vi "RegisterPublisher.vi"(6 "Lock Topic":bool, 7 "Topic Name":string, 8 "error in (no error)":errorcluster, 11 "Message Broker Interface Ref in":refnum<class "Message Broker Interface Ref.lvclass">) -> (0 "error out":errorcluster, 2 "Topic Actor Created?":bool, 3 "Message Broker Interface Ref out":refnum<class "Message Broker Interface Ref.lvclass">, 4 "Locked?":bool, 5 "Transport":refnum<class "Message Transport Queue.lvclass">)   [LabVIEW 2016, in "Stream Mediator.lvlib" / "Message Broker Interface Ref.lvclass"]
doc: "--\nCopyright © 2017 Composed SystemsI All rights reserved.\n\nAuthor: Jon McBee <jon.mcbee@composed.io>\n\nThis library is provided \"AS IS\" ,WITHOUT WARRANTIES OR\nCONDITIONS OF ANY KIND, either express or implied.\n\nComposed Systems -- composed.io\n\nStream 0.0.1.1\nJon McBee - Composed Systems\nCopyright (c) 2017, Composed Systems"
uses:
  <userlib>/Composed Systems/Stream/Mediator/Classes/Message Broker Interface Ref/Message Broker Interface Ref.lvclass
  <userlib>/Composed Systems/Stream/Mediator/Classes/Message Transport Queue/Message Transport Queue.lvclass
  <userlib>/Composed Systems/Stream/Mediator/Classes/Message Broker Interface Ref/Message Broker Interface Ref.lvclass/Message Broker Interface Ref.ctl
  <userlib>/Composed Systems/Stream/Mediator/Classes/Message Broker/Message Broker.lvclass
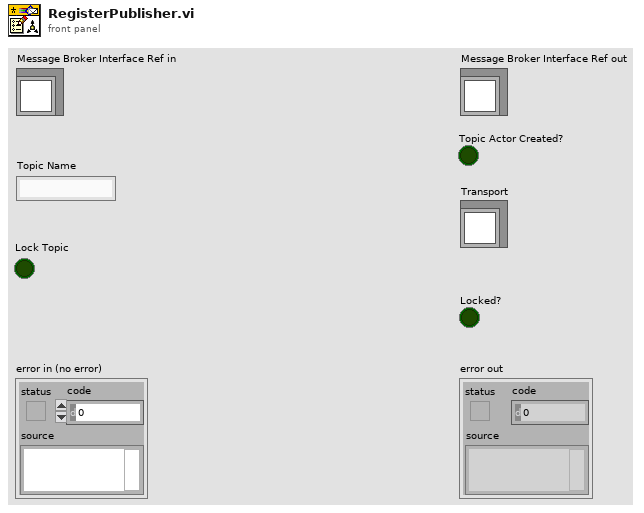
[diagram p1: front panel]
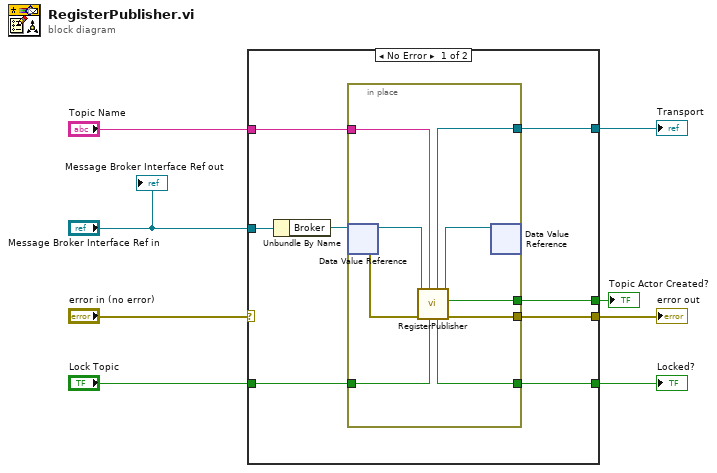
[diagram p0: block diagram]
diagram:
  n1 = case shown="No Error" "error in (no error)" {
    selector: "error in (no error)" -> [_ w26]
    tunnel: "Message Broker Interface Ref in" -> [w16 _]
    tunnel: "Topic Name" -> [w15 _]
    tunnel: "Lock Topic" -> [w14 _]
    tunnel: [w12 _] -> w4
    tunnel: [w11 w26] -> w3
    tunnel: [w10 _] -> w2
    tunnel: [w9 _] -> w1
    frame No Error {
      n2 = Unbundle By Name(w16) -> ("Broker"=w13:refnum<data-value>)
      n3 = in-place {
        in-place-border: w15 -> [w22]
        in-place-border: w14 -> [w21]
        in-place-border: [w20] -> w12
        in-place-border: [w19] -> w11
        in-place-border: [w18] -> w10
        in-place-border: [w17] -> w9
        n4 = in-place-dvr #1(w13) -> (w25:refnum<class "Message Broker.lvclass">, w23:errorcluster)
        n5 = call <userlib>:"RegisterPublisher.vi"("1:M"=w21, "Topic Name"=w22, "error in (no error)"=w23, "Message Broker in"=w25) -> ("error out"=w19:errorcluster, "Topic Actor Created?"=w17:bool, "Message Broker out"=w24:refnum<class "Message Broker.lvclass">, "Locked?"=w18:bool, "Transport"=w20:refnum<class "Message Transport Queue.lvclass">)  [unwired: 3 in]
        n6 = in-place-dvr #1(w24) -> ()  [unwired: 2 out]
      }
    }
    frame Error {
    }
  }
  "error out" <- w3
  "Transport" <- w4
  "Locked?" <- w2
  "Topic Actor Created?" <- w1
  "Message Broker Interface Ref out" <- "Message Broker Interface Ref in"
